vi "saturate float.vi"(8 "error in (no error)":errorcluster, 9 "max":sgl, 10 "min":sgl, 11 "val":sgl) -> (0 "error out":errorcluster, 2 "function return":i32, 3 "val out":sgl)   [LabVIEW 2014, in "test_IMU.lvlib"]
doc: "int saturate_float(float* val, float min, float max);"
uses:
  <userlib>/test_IMU/test_IMU.lvlib
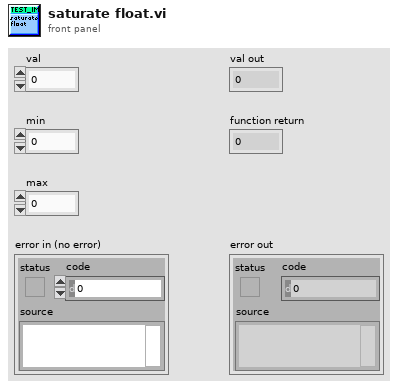
[diagram p1: front panel]
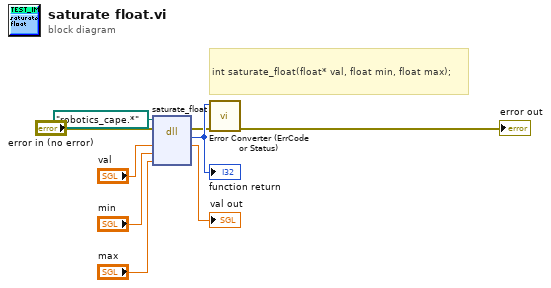
[diagram p0: block diagram]
diagram:
  # "int saturate_float(float* val, float min, float max);"
  n1 = dll-call lib="C:/Users/ktalke/Documents/Updated Header File/6.18.16/Compiled SO -schroot/robotics_cape.so" fn="saturate_float"(path in=path "robotics_cape.*", error in="error in (no error)", "val"="val", "min"="min", "max"="max") -> (error out=w3:errorcluster, "return type"=w9:i32, "val"=→"val out":sgl)  [unwired: 3 in, 1 out]
  "function return" <- w9
  n2 = call <userlib>:"Error Converter (ErrCode or Status).vi"("error in (no error)"=w3, "error code"=w9) -> ("error out"=→"error out":errorcluster)  [unwired: 9 in]
